vi "DC PS Control and Monitor.vi"() -> ()   [LabVIEW 2018]
uses:
  <vilib>/DAQmx/read.llb/DAQmx Read (Analog DBL 1Chan 1Samp).vi
  <vilib>/DAQmx/write.llb/DAQmx Write (Analog DBL 1Chan 1Samp).vi
  <vilib>/DAQmx/create/channels.llb/DAQmx Create Channel (AO-Voltage-Basic).vi
  <vilib>/DAQmx/create/channels.llb/DAQmx Create Channel (AI-Voltage-Basic).vi
  <vilib>/DAQmx/miscellaneous.llb/DAQmx Fill In Error Info.vi
  <vilib>/ptbypt/NI_PtbyPt.lvlib
panel:
  in  "y":dbl
  out "Control VDC":dbl
  in  "Slide":dbl(slide) min=0.0 max=36.0 step=0.5 scale=0.0..36.0
  out "Numeric 2":dbl format="%#.2g"
  out "Numeric":dbl
  out "error out 2":errorcluster
  out "error out":errorcluster
  out "Power Supply\nOutput VDC":dbl(knob) scale=0.0..36.0
  in  "Offset":dbl
  in  "Scale":dbl
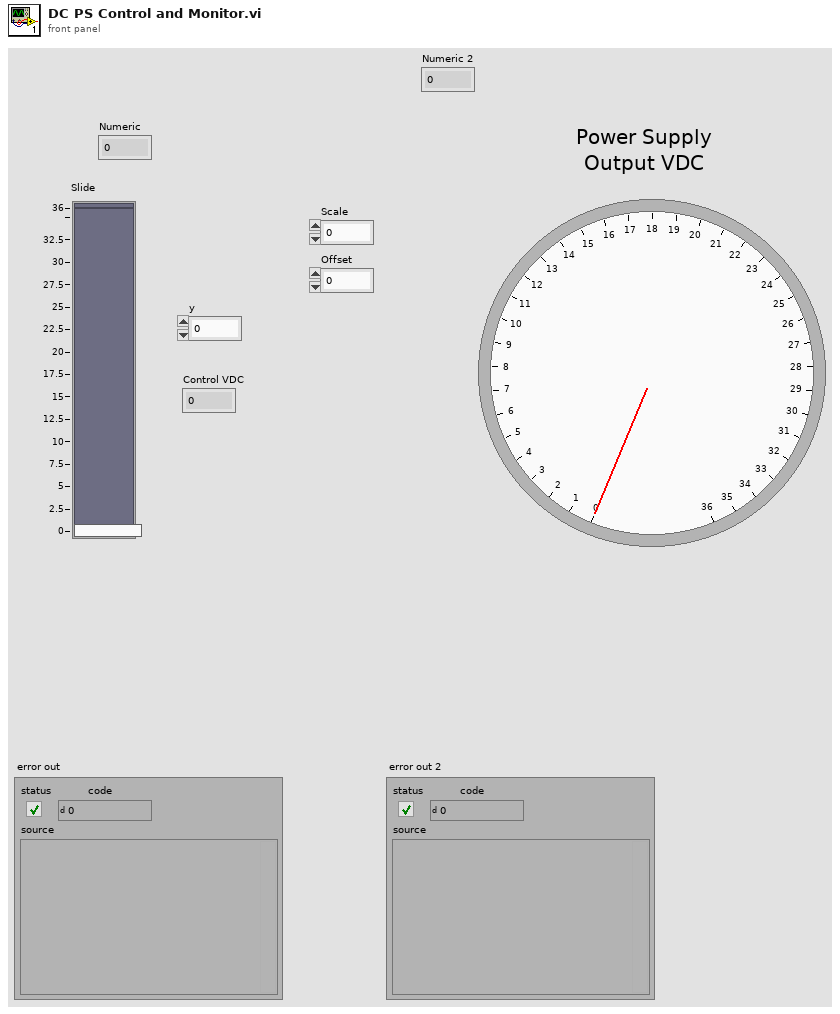
[diagram p1: front panel]
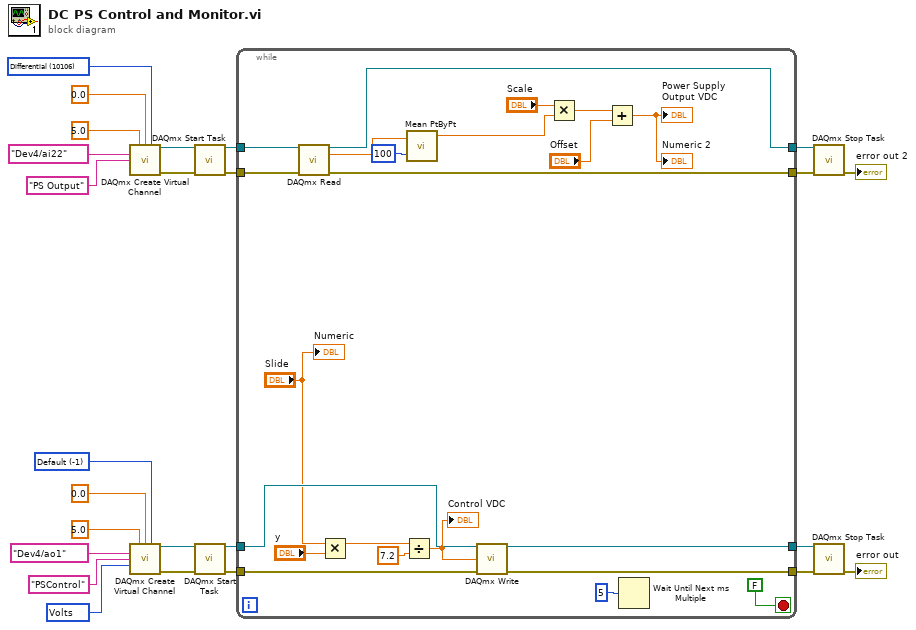
[diagram p0: block diagram]
diagram:
  w13 = 10106 items=["Default"=-1, "RSE"=10083, "NRSE"=10078, "Differential"=10106, "Pseudodifferential"=12529] ("input terminal configuration")
  w18 = -1 items=["Default"=-1, "RSE"=10083, "Differential"=10106, "Pseudodifferential"=12529] ("output terminal configuration")
  w23 = 10348 items=["Volts"=10348, "From Custom Scale"=10065] ("units")
  n1 = call-poly <vilib>:"DAQmx Create Virtual Channel.vi"("maximum value"=5.0, "minimum value"=0.0, "input terminal configuration"=w13, "physical channels"=tag "Dev4/ai22", "name to assign"="PS Output") -> ("task out"=w14:refnum<k21>, "error out"=w11:errorcluster)  [unwired: 9 in]
  n2 = call-poly <vilib>:"DAQmx Create Virtual Channel.vi"("maximum value"=5.0, "minimum value"=0.0, "output terminal configuration"=w18, "physical channels"=tag "Dev4/ao1", "name to assign"="PSControl", "units"=w23) -> ("task out"=w24:refnum<k21>, "error out"=w25:errorcluster)  [unwired: 8 in]
  n3 = call <vilib>:"DAQmx Start Task.vi"("task/channels in"=w14, "error in"=w11) -> ("task out"=w4:refnum<k21>, "error out"=w3:errorcluster)  [unwired: 12 in]
  n4 = call <vilib>:"DAQmx Start Task.vi"("task/channels in"=w24, "error in"=w25) -> ("task out"=w10:refnum<k21>, "error out"=w9:errorcluster)  [unwired: 12 in]
  n5 = while {
    tunnel: w10 -> [w46]
    tunnel: w9 -> [w45]
    tunnel: [w44] -> w6
    tunnel: [w43] -> w5
    tunnel: w4 -> [w42]
    tunnel: w3 -> [w41]
    tunnel: [w37] -> w2
    tunnel: [w36] -> w1
    stop <- FALSE stop-if-true
    n6 = call-poly <vilib>:"DAQmx Read.vi"("task/channels in"=w42, "error in"=w41) -> ("task out"=w37:refnum<k21>, "data"=w33:dbl, "error out"=w36:errorcluster)  [unwired: 11 in]
    n7 = Multiply(x="Slide", y="y") -> (x*y=w27:dbl)
    n8 = Divide(x=w27, y=7.2) -> (x/y=w28:dbl)
    "Control VDC" <- w28
    n9 = call <vilib>:"Mean PtByPt.vi"("x"=w33, "sample length"=100) -> ("mean"=w32:dbl)  [unwired: 2 in, 1 out]
    n10 = call-poly <vilib>:"DAQmx Write.vi"("task/channels in"=w46, "data"=w28, "error in"=w45) -> ("task out"=w44:refnum<k21>, "error out"=w43:errorcluster)  [unwired: 10 in, 1 out]
    n11 = Multiply(x="Scale", y=w32) -> (x*y=w38:dbl)
    n12 = Add(x=w38, y="Offset") -> (x+y=→"Power Supply\nOutput VDC" →"Numeric 2":dbl)
    n13 = Wait Until Next ms Multiple(millisecond multiple=u32 5) -> ()  [unwired: 1 out]
    "Numeric" <- "Slide"
  }
  n14 = call <vilib>:"DAQmx Stop Task.vi"("task/channels in"=w2, "error in"=w1) -> ("error out"=→"error out 2":errorcluster)  [unwired: 12 in, 1 out]
  n15 = call <vilib>:"DAQmx Stop Task.vi"("task/channels in"=w6, "error in"=w5) -> ("error out"=→"error out":errorcluster)  [unwired: 12 in, 1 out]
